vi "Inst.Transport.Public API.vi"(8 "error in (no error)":errorcluster, 11 "Instrument.Transport in":refnum<class "Inst.Transport.lvclass">) -> (0 "error out":errorcluster, 2 "commands (this level)":string[](array[string]), 3 "Instrument.Transport out":refnum<class "Inst.Transport.lvclass">)   [LabVIEW 2019, in "Inst.Transport.lvclass"]
doc: "Override this VI to return a list of commands only supported by your Instrument"
uses:
  Inst.Transport.lvclass
  Typedefs/Inst.Transport.PublicCommands--Enum.ctl
  e1de43f0-20b4-4b68-9ad7-6af06000068d.vi
  <vilib>/Utility/Data Type/Get Type Information.vi
  <vilib>/Utility/Data Type/Get Numeric Information.vi
  <userlib>/_OpenG.lib/lvdata/lvdata.llb/Unwrap VVariant__ogtk.vi
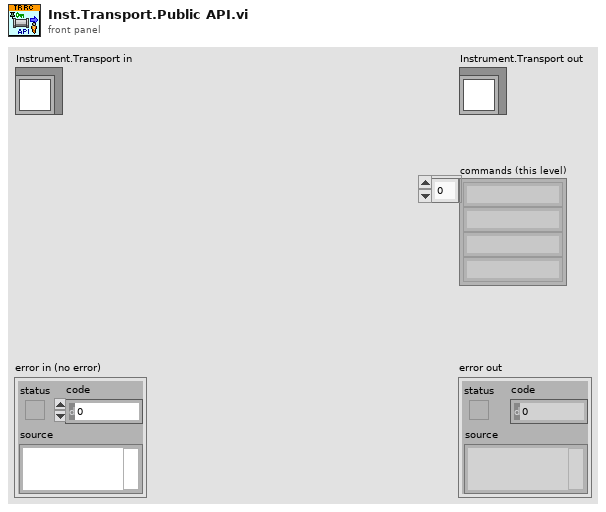
[diagram p1: front panel]
types:
  T1 = typedef "Inst.Transport.lvclass/Inst.Transport.PublicCommands--Enum.ctl" = enum16{"doSomething"}
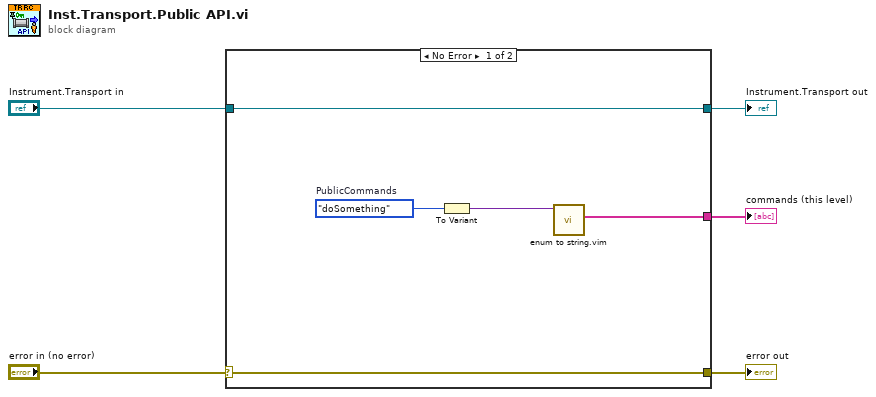
[diagram p0: block diagram]
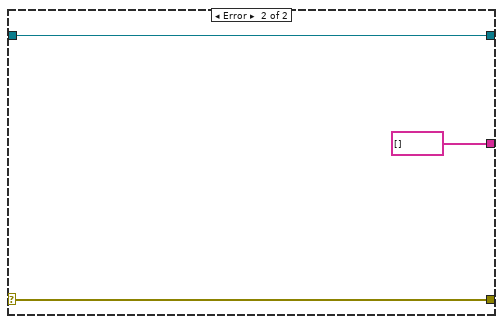
[diagram p2: hidden frame]
diagram:
  n1 = case shown="No Error" "error in (no error)" {
    selector: "error in (no error)" -> [w8 w13]
    tunnel: [w8 w13] -> w4
    tunnel: [w9 w12] -> w1
    tunnel: "Instrument.Transport in" -> [w9 w12]
    tunnel: [w10 string[] [] ("Array")] -> w2
    frame No Error {
      w6 = Inst.Transport.PublicCommands--Enum."doSomething"  # PublicCommands
      n2 = To Variant(anything=w6) -> (Variant=w7:variant)
      n3 = call "enum to string.vim"("enum in"=w7) -> ("strings out"=w10:string[])  [unwired: 9 in, 1 out]
    }
    frame Error {
    }
  }
  "error out" <- w4
  "Instrument.Transport out" <- w1
  "commands (this level)" <- w2
